vi "URAPI_WriteCOMOut_num.vi"(0 "Variable In":string="line", 3 "URAPI Script":T1={"Script"="", "Whiles"=[], "Ifs"=[], "Supress Err"=TRUE, "Errors"=""}, 4 "Port":u8) -> (2 "Variable Out":string, 5 "URAPI Script":T1={"Script"="", "Whiles"=[], "Ifs"=[], "Supress Err"=TRUE, "Errors"=""})   [LabVIEW 2012]
doc: "Writes the value of \"Variable In\" to the specified COM \"Port\"."
uses:
  <userlib>/BotSpeak/VIs/Direct/URAPI_Control.ctl
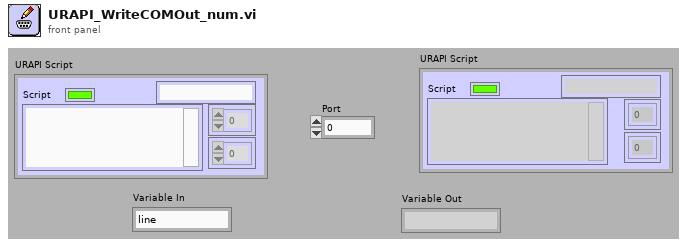
[diagram p1: front panel]
types:
  T1 = typedef "URAPI_Control.ctl" = cluster{"Script":string, "Whiles":u8[], "Ifs":u8[], "Supress Err":bool, "Errors":string}
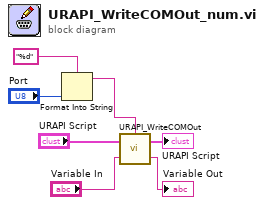
[diagram p0: block diagram]
diagram:
  n1 = Format Into String(format string="%d" ("string"), "Port") -> (resulting string=w1:string)  [unwired: 2 in, 1 out]
  n2 = call <userlib>:"URAPI_WriteCOMOut.vi"("Variable In"="Variable In", "URAPI Script"="URAPI Script", "Port"=w1) -> ("Variable Out"=→"Variable Out":string, "URAPI Script"=→"URAPI Script":T1)  [unwired: 1 in]
